vi "Size1001.vi"   [LabVIEW 2013]
uses:
  <vilib>/Heliosphere Research LLC/Advanced Plotting Toolkit/Advanced Plotting Toolkit.lvlib
types:
  T1 = typedef "Advanced Plotting Toolkit.lvlib/PlotID.ctl" = i32
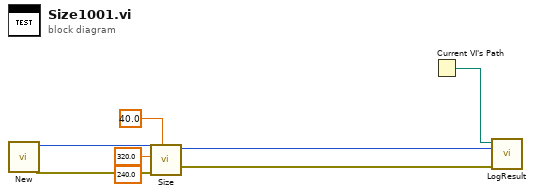
[diagram p0: block diagram]
diagram:
  n1 = call <vilib>:"New.vi"() -> ("error out"=w4:errorcluster, "Plot ID"=w7:T1)  [unwired: 10 in]
  n2 = call <vilib>:"Size.vi"("DPI"=40.0, "error in (no error)"=w4, "Height (pixels)"=240.0, "Width (pixels)"=320.0, "Plot ID"=w7) -> ("error out"=w5:errorcluster, "Plot ID Out"=w6:T1)  [unwired: 5 in]
  n3 = Current VI's Path() -> (path=w8:path)
  n4 = call "LogResult.vi"("Test Result"=w5, "Test Artifact"=w6, "VI Path"=w8) -> ()  [unwired: 9 in]
